vi "ForTest.vi"(8 "error in (no error)":errorcluster) -> (0 "error out":errorcluster, 3 "Color Out":u32(colorbox))   [LabVIEW 2015]
panel:
  in  "stop":bool
  in  "Color Box":u32(colorbox)
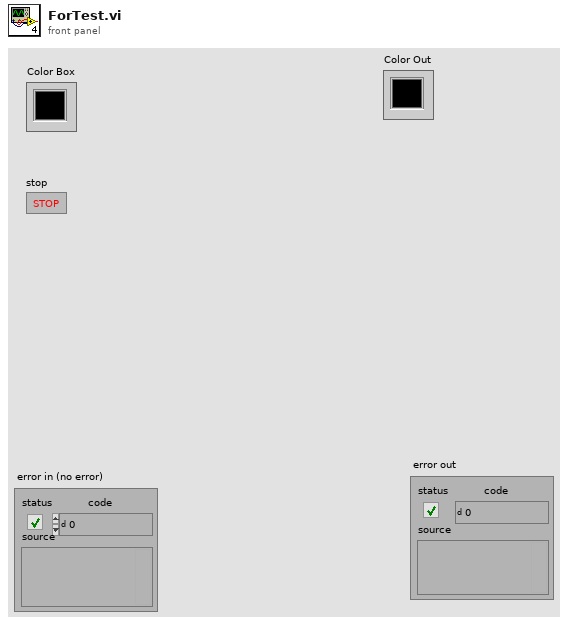
[diagram p1: front panel]
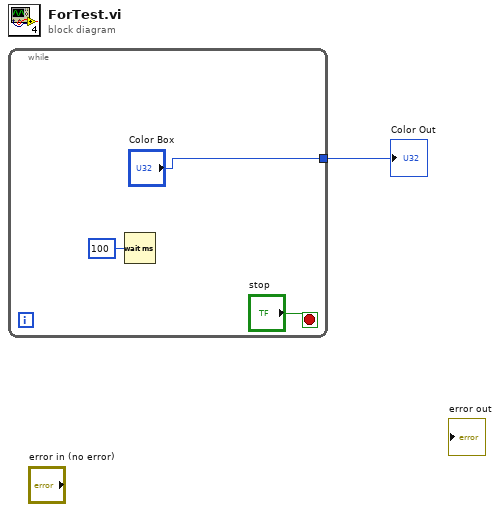
[diagram p0: block diagram]
diagram:
  n1 = while {
    tunnel: ["Color Box"] -> w1
    stop <- "stop" stop-if-true
    n2 = Wait (ms)(milliseconds to wait=u32 100) -> ()  [unwired: 1 out]
  }
  "Color Out" <- w1
